vi "CalibrationDueWarning.vi"() -> (1 "Message":string, 2 "Traffic Light":cluster{"Red":bool, "Amber":bool, "Green":bool} caption="Calibration Status")   [LabVIEW 2017, in "CalibrationManagerActor.lvlib" / "CalibrationManagerActor.lvclass"]
uses:
  CalibrationManagerActor.lvclass
  SAMLite_DB/DB_Collections_class/mode.ctl
  SAMLite_DB/DB_Collections_class/DB_Collections.lvclass
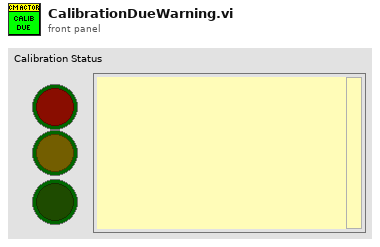
[diagram p1: front panel]
types:
  T1 = typedef "SAMLite_DB.lvlib/DB_Collections.lvclass/mode.ctl" = enum16{"read from file", "write to file", "set Defaults"}
  T2 = typedef "SAMLite_DB.lvlib/DB_Collections.lvclass/SAMLite Database.ctl" = cluster{"User Management":T3, "File Paths":cluster{"Path of test modules":path, "Path of sequences":path, "Path of test reports":path, "Path of Error Report":path, "Path of Calibration Data File":path, "Path of Company Logo":path, "Path of Startup VIs":path}, "Version Info":cluster{"Version No.":string}, "GUI Configuration":T6, "TARTCS_Intrument Control":T7, "Step Module Data":T15}
  T3 = typedef "SAMLite_DB.lvlib/DB_User.lvclass/User Management.ctl" = cluster{"Current User":string, "Current user group":T4, "Registered Users":cluster{"First Name":string, "Last Name":string, "User Name":string, "Password":string, "User Group":T4}[], "User Groups":cluster{"User Group":T4, "Members":string[], "User Previleges":T5}[]}
  T4 = typedef "SAMLite_DB.lvlib/DB_User.lvclass/User Group.ctl" = enum16{"Administrator", "Engineer", "Operator", "Data Viewer"}
  T5 = typedef "SAMLite_DB.lvlib/DB_User.lvclass/User Previleges.ctl" = cluster{"Run Sequences":bool, "Set Station Options":bool, "Instrument Configurations":bool, "Calibration Management":bool, "Access Test Reports Screen":bool, "Edit Test Sequences":bool, "Edit User":bool, "Add User":bool, "Delete User":bool, "Manual Control":bool, "Initialise System":bool}
  T6 = typedef "SAMLite_DB.lvlib/DB_SoftConfig.lvclass/GUI_Configurations.ctl" = cluster{"Main screen button caption color":u32, "Main screen display setting":enum32{"Modal", "Floating"}, "Debug Mode?":bool}
  T7 = typedef "SAMLite_DB.lvlib/DB_Collections.lvclass/TARTCS_InstrumentsSettings.ctl" = cluster{"Boom":T8, "Turntable":T11, "Inclinometer":T12, "Signal Generator Settings":cluster{"Resource Name (GPIB::28)":string}, "Spectrum Analyser Settings":cluster{"Resource Name (GPIB::28)":string}, "cRIO IP address":cluster{"Resource Name (GPIB::28)":string}}
  T8 = typedef "StreamComms.lvlib/Boom_Params.ctl" = cluster{"Master Node detail ":T9, "Slave Node Detail":T9, "Angle":dbl, "Motor Frequency %":dbl, "Max Leg Angle Difference":dbl, "Max Inclinometer to To Boom Leg  Angle Difference":dbl, "Angle Limits":cluster{"Max Operating Position":dbl, "Home Max Offset":dbl, "Home Position":dbl, "Home Min Offset":dbl, "Min Operating Position":dbl}, "Step Angle":dbl, "Select Boom/Inc Trigger":enum16{"Inclinometer", "Boom"}}
  T9 = typedef "StreamComms.lvlib/Inverter_NodeInfo.ctl" = cluster{"Node ID":u8, "baud rate":T10, "termination required? (F)":bool, "interface name":u32, "Inverter Name":string}
  T10 = typedef "CANopen BaudRate.ctl" = u32
  T11 = typedef "StreamComms.lvlib/Turntable_Params.ctl" = cluster{"Node Detail":T9, "Angle":dbl, "Motor Frequency %":dbl, "Trigger Step Angle":dbl}
  T12 = typedef "StreamComms.lvlib/Inclinometer_Params.ctl" = cluster{"Node Detail":T13, "filter cutoff (milli Hz)":dbl, "Triger angle":dbl, "Zero Offset (deg)":dbl}
  T13 = typedef "StreamComms.lvlib/CANOpen_NodeDetail.ctl" = cluster{"LSS Identity Details":T14, "Node ID":u8, "baud rate":T10, "termination required? (F)":bool, "interface name":u32}
  T14 = typedef "StreamComms.lvlib/CANOpen LSS Identity.ctl" = cluster{"Vendor ID":u32, "Product Code":u32, "Revision Number":u32, "Serial Number":u32}
  T15 = typedef "SAMLite_DB.lvlib/DB_StepModule.lvclass/Step Module Date.ctl" = cluster{"Error Out":errorcluster}
  T16 = typedef "SAMLite_Calibration Managemer.lvlib/CalManData.ctl" = cluster{"Cal Warning":u32, "Cnt Warning":u16, "Cal Data Listing":T17[]}
  T17 = typedef "SAMLite_Calibration Managemer.lvlib/CalDataUnit.ctl" = cluster{"Alias":string, "Description":string, "S/N":string, "Type":string, "Cal Date":timestamp, "Cal Due":timestamp, "Cal Data File":path, "Total Cycles":i32, "Cycles Elapsed":i32}
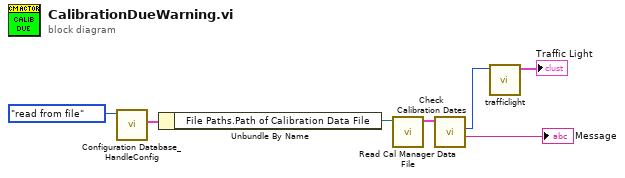
[diagram p0: block diagram]
diagram:
  n1 = call "Configuration Database_HandleConfig.vi"("Task"=mode."read from file") -> ("SAMLite Database  out"=w5:T2)  [unwired: 9 in, 1 out]
  n2 = Unbundle By Name(w5) -> ("File Paths.Path of Calibration Data File"=w3:path)
  n3 = call "Read Cal Manager Data File.vi"("Calibration File"=w3) -> ("Calibration Data"=w2:T16)  [unwired: 9 in, 1 out]
  n4 = call "Check Calibration Dates.vi"("Calibration Data"=w2) -> ("Message Out"=→"Message":string, "Status"=w1:u16)  [unwired: 7 in, 2 out]
  n5 = call "trafficlight.vi"("Status"=w1) -> ("Traffic Light"=→"Traffic Light":cluster{"Red":bool, "Amber":bool, "Green":bool})  [unwired: 7 in]
